vi "Check If Arrays Equal.vi"(4 "y":u8[](array[numeric])=[0, 0, 0, 0, 0, 0, 0, 0, 0, 0, 0, 0], 5 "x":u8[](array[numeric])=[0, 0, 0, 0, 0, 0, 0, 0, 0, 0, 0, 0]) -> (1 "x != y?":bool)   [LabVIEW 2019]
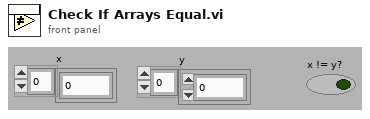
[diagram p1: front panel]
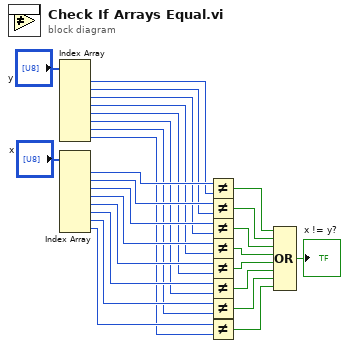
[diagram p0: block diagram]
diagram:
  n1 = Index Array(array="y") -> (element #1=w24:u8, element #2=w22:u8, element #3=w15:u8, element #4=w14:u8, element #5=w13:u8, element #6=w12:u8, element #7=w11:u8, element #8=w10:u8)  [unwired: 8 in]
  n2 = Index Array(array="x") -> (element #1=w25:u8, element #2=w23:u8, element #3=w21:u8, element #4=w20:u8, element #5=w19:u8, element #6=w18:u8, element #7=w17:u8, element #8=w16:u8)  [unwired: 8 in]
  n3 = Not Equal?(x=w25, y=w24) -> (x != y?=w9:bool)
  n4 = Not Equal?(x=w23, y=w22) -> (x != y?=w8:bool)
  n5 = Not Equal?(x=w21, y=w15) -> (x != y?=w7:bool)
  n6 = Not Equal?(x=w20, y=w14) -> (x != y?=w6:bool)
  n7 = Not Equal?(x=w19, y=w13) -> (x != y?=w5:bool)
  n8 = Not Equal?(x=w18, y=w12) -> (x != y?=w1:bool)
  n9 = Not Equal?(x=w17, y=w11) -> (x != y?=w4:bool)
  n10 = Not Equal?(x=w16, y=w10) -> (x != y?=w3:bool)
  n11 = Compound Arithmetic op=OR(w9, w8, w7, w6, w5, w1, w4, w3) -> (→"x != y?":bool)
